vi "Initialize_Stack_Autorange.vi"(0 "2182A VISA in":refnum<visa-resource-name>, 1 "21282A Error In":errorcluster, 2 "6221 VISA in":refnum<visa-resource-name>, 3 "Compliance (V)":dbl, 4 "Output Response":bool, 5 "6221 Error In":errorcluster) -> (14 "2182A VISA out":refnum<visa-resource-name>, 15 "2182A Error Out":errorcluster, 16 "6221 VISA out":refnum<visa-resource-name>, 19 "6221 Error Out":errorcluster)   [LabVIEW 2014]
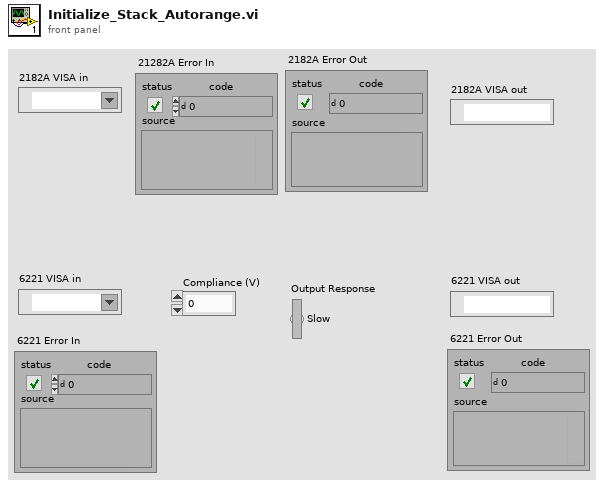
[diagram p1: front panel]
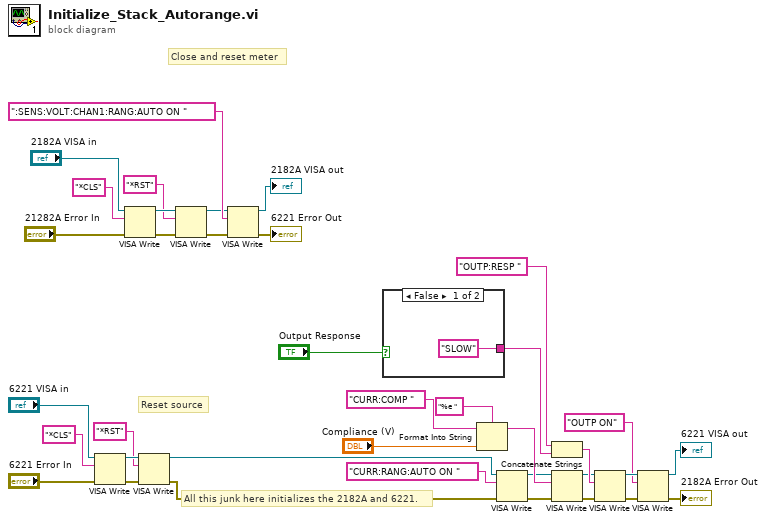
[diagram p0: block diagram]
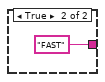
[diagram p2: hidden frame]
diagram:
  # "All this junk here initializes the 2182A and 6221."
  # "Reset source"
  # "Close and reset meter"
  n1 = VISA Write(VISA resource name="6221 VISA in", write buffer="*CLS", error in (no error)="6221 Error In") -> (VISA resource name out=w37:refnum<visa-resource-name>, error out=w36:errorcluster)  [unwired: 1 out]
  n2 = VISA Write(VISA resource name="2182A VISA in", write buffer="*CLS", error in (no error)="21282A Error In") -> (VISA resource name out=w34:refnum<visa-resource-name>, error out=w31:errorcluster)  [unwired: 1 out]
  n3 = VISA Write(VISA resource name=w37, write buffer="*RST", error in (no error)=w36) -> (VISA resource name out=w8:refnum<visa-resource-name>, error out=w7:errorcluster)  [unwired: 1 out]
  n4 = VISA Write(VISA resource name=w34, write buffer="*RST", error in (no error)=w31) -> (VISA resource name out=w10:refnum<visa-resource-name>, error out=w9:errorcluster)  [unwired: 1 out]
  n5 = VISA Write(VISA resource name=w10, write buffer=":SENS:VOLT:CHAN1:RANG:AUTO ON ", error in (no error)=w9) -> (VISA resource name out=→"2182A VISA out":refnum<visa-resource-name>, error out=→"6221 Error Out":errorcluster)  [unwired: 1 out]
  n6 = case shown="False" "Output Response" {
    tunnel: ["SLOW" "FAST"] -> w18
    frame False {
    }
    frame True {
    }
  }
  n7 = Format Into String(format string="%e ", initial string="CURR:COMP ", "Compliance (V)") -> (resulting string=w20:string)  [unwired: 1 in, 1 out]
  n8 = VISA Write(VISA resource name=w8, write buffer="CURR:RANG:AUTO ON ", error in (no error)=w7) -> (VISA resource name out=w15:refnum<visa-resource-name>, error out=w14:errorcluster)  [unwired: 1 out]
  n9 = Concatenate Strings("OUTP:RESP ", w18) -> (w16:string)
  n10 = VISA Write(VISA resource name=w15, write buffer=w20, error in (no error)=w14) -> (VISA resource name out=w12:refnum<visa-resource-name>, error out=w13:errorcluster)  [unwired: 1 out]
  n11 = VISA Write(VISA resource name=w12, write buffer=w16, error in (no error)=w13) -> (VISA resource name out=w24:refnum<visa-resource-name>, error out=w25:errorcluster)  [unwired: 1 out]
  n12 = VISA Write(VISA resource name=w24, write buffer="OUTP ON", error in (no error)=w25) -> (VISA resource name out=→"6221 VISA out":refnum<visa-resource-name>, error out=→"2182A Error Out":errorcluster)  [unwired: 1 out]
